vi "Configure Math Reading.vi"(0 "VISA resource name":refnum<visa-resource-name>, 1 "Enable Math Reading (F: Disable)":bool, 5 "Math Calculation (0: Linear)":u16(ring) items=["Linear", "Reciprocal", "Logarithmic"], 7 "Scale Factor (1.0)":dbl=1.0, 9 "Linear Offset (0)":dbl, 11 "error in (no error)":errorcluster) -> (4 "VISA resource name out":refnum<visa-resource-name>, 15 "error out":errorcluster)   [LabVIEW 2021, in "Keithley 648X Series.lvlib"]
doc: "Configures the math reading calculation. \n\n<b>Note:</b>\nThe math calculation applies to the reading output of the filters. If these raw readings are desired use the linear math calculation with a scale factor of 1 and offset of 0."
uses:
  <instrlib>/Keithley 648X Series/Keithley 648X Series.lvlib
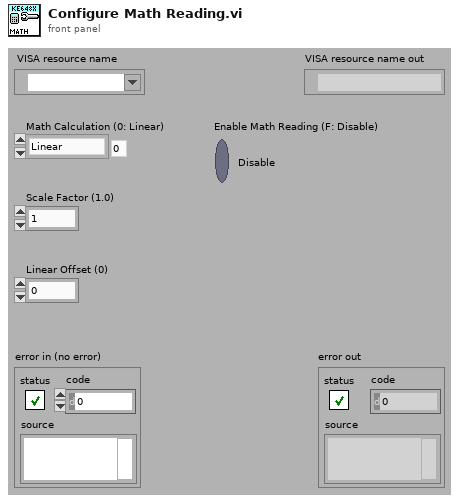
[diagram p1: front panel]
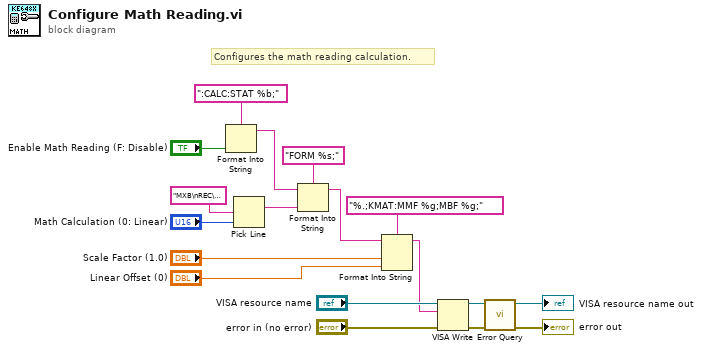
[diagram p0: block diagram]
diagram:
  # "Configures the math reading calculation."
  n1 = Format Into String(format string=":CALC:STAT %b;", "Enable Math Reading (F: Disable)") -> (resulting string=w6:string)  [unwired: 2 in, 1 out]
  n2 = Pick Line(multi-line string="MXB\nREC\nLOG10", line index="Math Calculation (0: Linear)") -> (output string=w9:string)  [unwired: 1 in]
  n3 = Format Into String(format string="FORM %s;", initial string=w6, w9) -> (resulting string=w2:string)  [unwired: 1 in, 1 out]
  n4 = Format Into String(format string="%.;KMAT:MMF %g;MBF %g;", initial string=w2, "Scale Factor (1.0)", "Linear Offset (0)") -> (resulting string=w1:string)  [unwired: 1 in, 1 out]
  n5 = VISA Write(VISA resource name="VISA resource name", write buffer=w1, error in (no error)="error in (no error)") -> (VISA resource name out=w14:refnum<visa-resource-name>, error out=w13:errorcluster)  [unwired: 1 out]
  n6 = call <instrlib>:"Error Query.vi"("error in (no error)"=w13, "VISA resource name"=w14) -> ("error out"=→"error out":errorcluster, "VISA resource name out"=→"VISA resource name out":refnum<visa-resource-name>)  [unwired: 6 in, 2 out]
